vi "set time to remote controller.vi"() -> ()   [LabVIEW 2019]
uses:
  <vilib>/nisyscfg/nisyscfg.lvlib
panel:
  out "Detailed Result":string
  out "error out":errorcluster
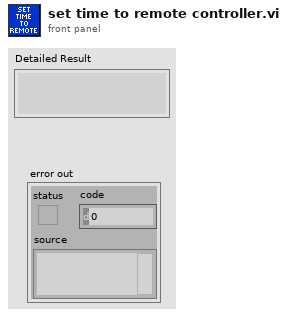
[diagram p1: front panel]
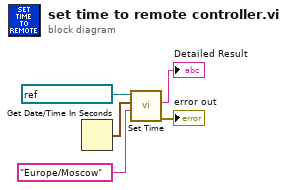
[diagram p0: block diagram]
diagram:
  n1 = Get Date/Time In Seconds() -> (seconds since 1Jan1904=w4:timestamp)
  n2 = call <vilib>:"Set Time.vi"("Time Zone"="Europe/Moscow", "Time"=w4, "Session in (localhost)"=refnum<k21> "192.168.1.10") -> ("error out"=→"error out":errorcluster, "Detailed Result"=→"Detailed Result":string)  [unwired: 5 in, 2 out]
